vi "SetSize.vi"(8 "size":i32, 11 "SubChannel in":refnum<class "SubChannelCPU.lvclass">) -> (3 "SubChannel out":refnum<class "SubChannelCPU.lvclass">)   [LabVIEW 2019, in "MessengerM.lvlib" / "SubChannelCPU.lvclass"]
uses:
  SubChannelCPU.lvclass
  <resource>/ChannelSupport/_ChannelSupport/PipeLogic2/PipeLogic2.lvclass
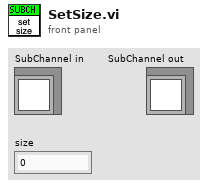
[diagram p1: front panel]
types:
  T1 = typedef "MessengerM.lvlib/Element.ctl" = string
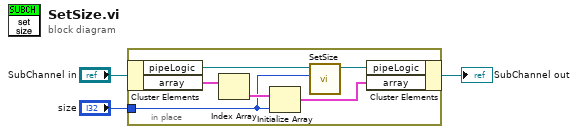
[diagram p0: block diagram]
diagram:
  n1 = in-place {
    in-place-border: "size" -> [w4]
    n2 = in-place-cluster #1("SubChannel in") -> ("pipeLogic"=w6:refnum<class "PipeLogic2.lvclass">, "array"=w9:cluster{"elt":T1}[])
    n3 = Index Array(array=w9) -> (element=w8:cluster{"elt":T1})  [unwired: 1 in]
    n4 = Initialize Array(w8, w4) -> (w7:cluster{"elt":T1}[])
    n5 = call <resource>:"SetSize.vi"("size"=w4, "pipeLogic in"=w6) -> ("pipeLogic out"=w5:refnum<class "PipeLogic2.lvclass">)  [unwired: 9 in]
    n6 = in-place-cluster #1("pipeLogic"=w5, "array"=w7) -> (→"SubChannel out":refnum<class "SubChannelCPU.lvclass">)
  }
